vi "Delete Int32Array DVR.vi"(8 "error in (no error)":errorcluster, 11 "Int32Array DVR in":refnum<data-value>) -> (0 "error out":errorcluster, 3 "Int32Array out":refnum<class "Int32Array.lvclass">)   [LabVIEW 2015, in "MDSplus.lvlib" / "Int32Array.lvclass"]
uses:
  <vilib>/MDSplus/Classes/Data_Class/Array_Class/Int32Array_Class/Int32Array.lvclass
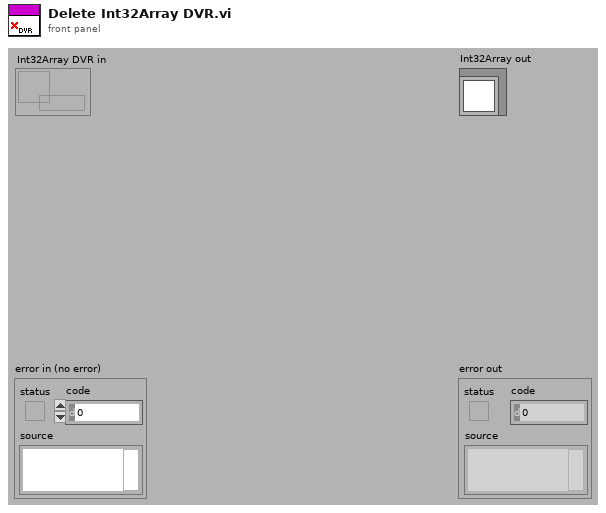
[diagram p1: front panel]
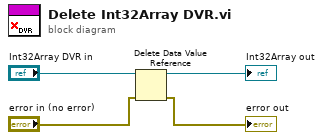
[diagram p0: block diagram]
diagram:
  n1 = Delete Data Value Reference(data value reference="Int32Array DVR in", error in="error in (no error)") -> (data value=→"Int32Array out":refnum<class "Int32Array.lvclass">, error out=→"error out":errorcluster)
